vi "GSP_Piezo_GUI.vi"(4 "error in (no error)":errorcluster) -> (0 "error out":errorcluster, 1 "Canceled?":bool, 2 "Piezo Setpoints":T1)   [LabVIEW 2015]
uses:
  piezo_setpoint.ctl
  GSP_CF_Global.vi
panel:
  in  "OK Button":bool
  in  "Right Piezo":i32
  in  "Left Piezo":i32
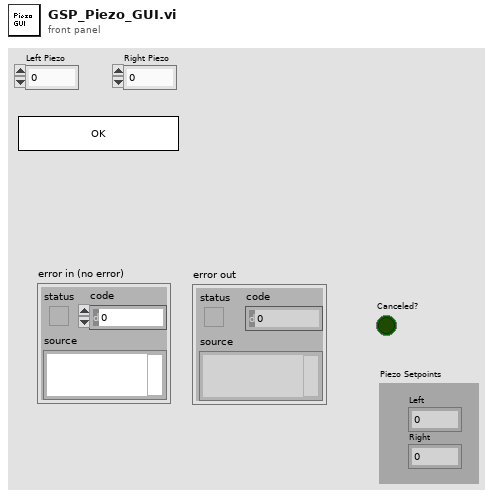
[diagram p1: front panel]
types:
  T1 = typedef "piezo_setpoint.ctl" = cluster{"Left":i32, "Right":i32}
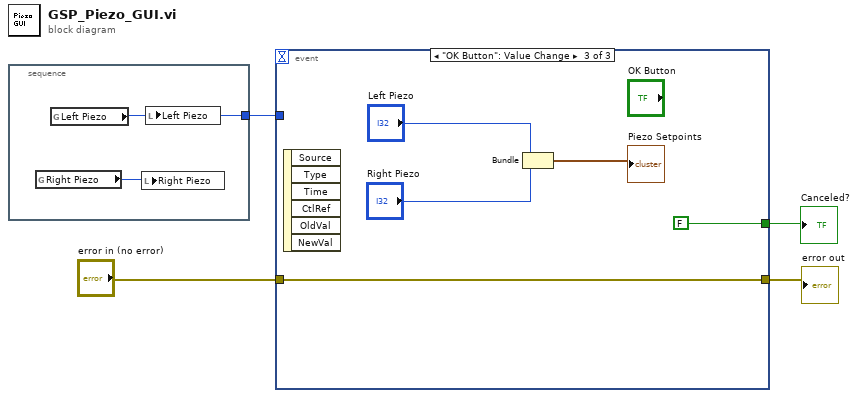
[diagram p0: block diagram]
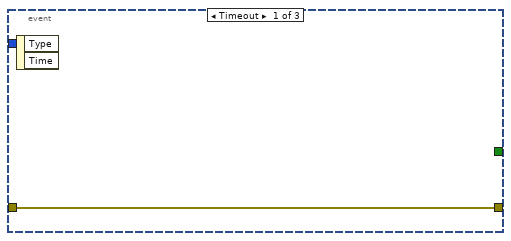
[diagram p2: hidden frame]
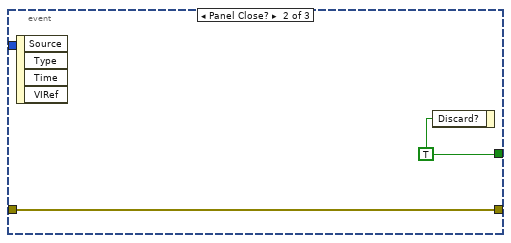
[diagram p3: hidden frame]
diagram:
  n1 = stacked-sequence {
    tunnel: [w5] -> w1
    frame #0 {
      n2 = global read "GSP_CF_Global.vi" "Right Piezo"() -> (w6:i32)
      n3 = global read "GSP_CF_Global.vi" "Left Piezo"() -> (w5:i32)
      n4 = local write "Right Piezo"(w6) -> ()
      n5 = local write "Left Piezo"(w5) -> ()
    }
  }
  n6 = event shown="[2] \"OK Button\": Value Change" {
    selector: _ -> [_ _ _]
    dyn-events: _ -> [_ _ _]
    timeout: _ -> [_ _ _]
    tunnel: [_ w9 FALSE] -> w4
    tunnel: "error in (no error)" -> [w7 w8 w10]
    tunnel: [w7 w8 w10] -> w3
    tunnel: w1 -> [_ _ _]
    event Timeout {
      n7 = event-data() -> ()  [unwired: 1 in, 2 out]
    }
    event Panel Close? {
      w9 = TRUE
      n8 = event-data() -> ()  [unwired: 1 in, 4 out]
      n9 = event-data("Discard?"=w9) -> ()  [unwired: 1 in, 1 out]
    }
    event "OK Button": Value Change {
      n10 = event-data() -> ()  [unwired: 1 in, 6 out]
      n11 = Bundle("Left Piezo"="Left Piezo", "Right Piezo"="Right Piezo") -> (→"Piezo Setpoints":cluster{"Left Piezo":i32, "Right Piezo":i32})  [unwired: 1 in]
    }
  }
  "Canceled?" <- w4
  "error out" <- w3
